vi "Main VI.vi"() -> ()   [LabVIEW 2020]
uses:
  Type Def - States Machine.ctl
  <vilib>/Instr/_visa.llb/VISA Configure Serial Port (Instr).vi
panel:
  in  "Start":bool
  in  "Bytes to read":u32
  out "Chart - Humidity":dbl(graph)
  out "Chart - Temperature":dbl(graph)
  in  "stop":bool
  in  "File Path":path
  in  "Time before receiving data (Seconds)":dbl
  out "Humidity (%)":dbl
  out "Temperature":dbl
  in  "Separator Term":string
  in  "Command Letter":string
  in  "Connection port":refnum<visa-resource-name>
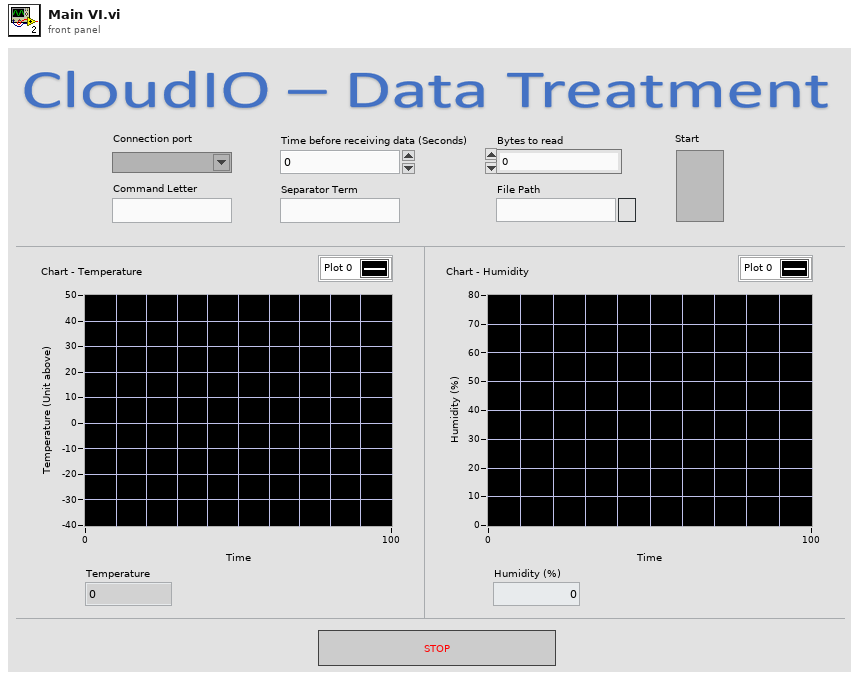
[diagram p1: front panel]
types:
  T1 = typedef "Type Def - States Machine.ctl" = enum16{"Idle", "Open Serial", "Request", "Receive", "Recording", "Close Serial"}
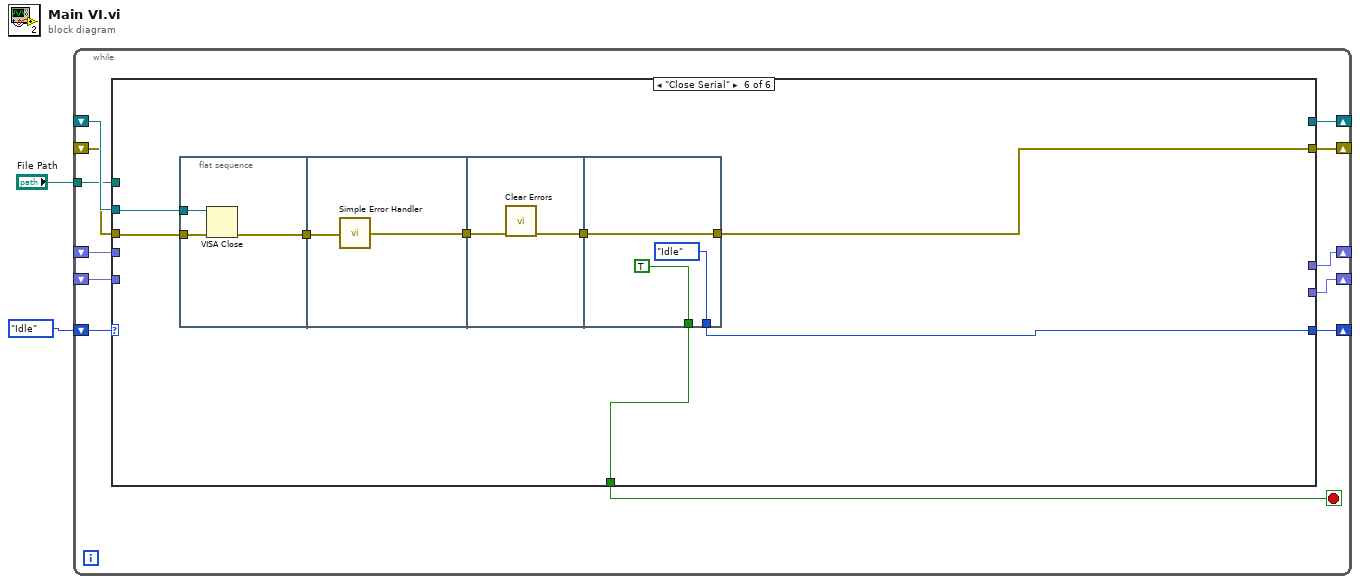
[diagram p0: block diagram]
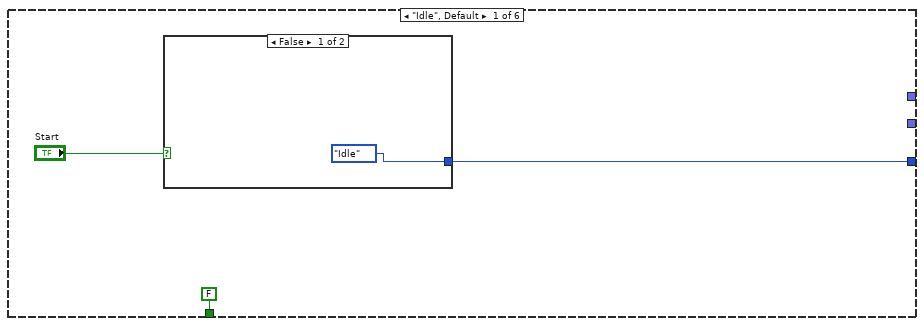
[diagram p2: hidden frame]
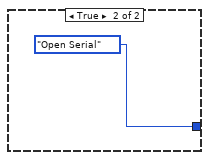
[diagram p3: hidden frame]
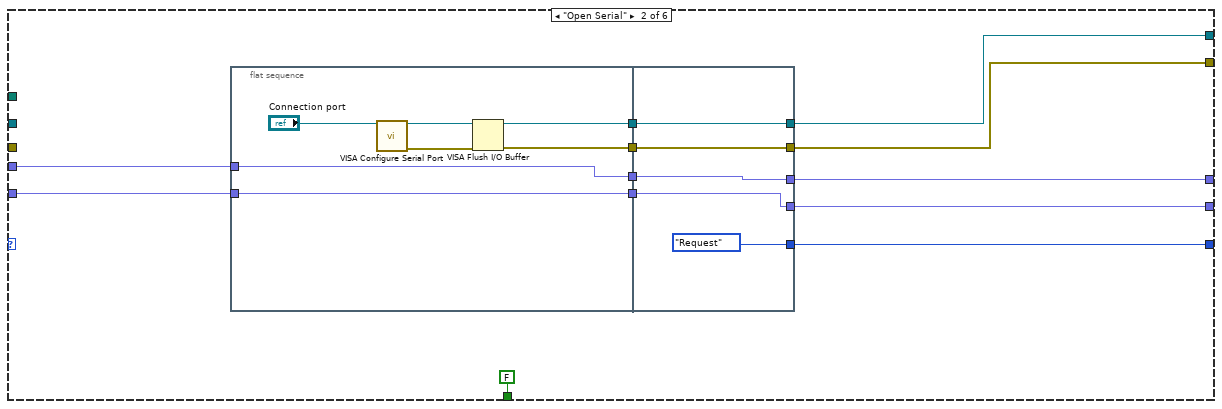
[diagram p4: hidden frame]
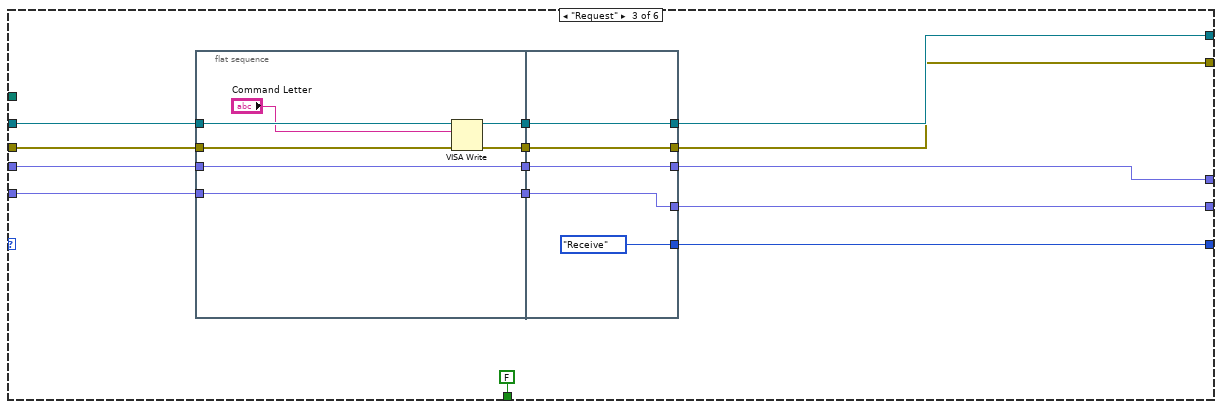
[diagram p5: hidden frame]
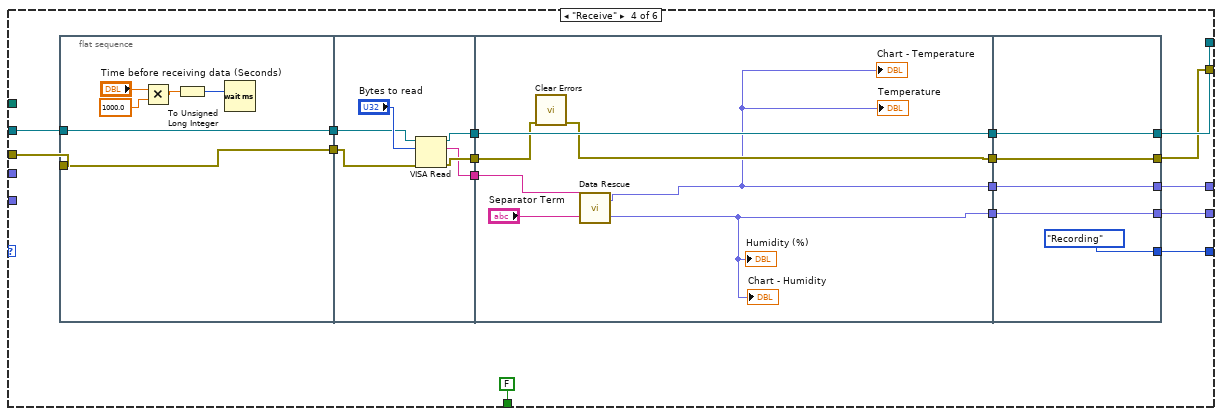
[diagram p6: hidden frame]
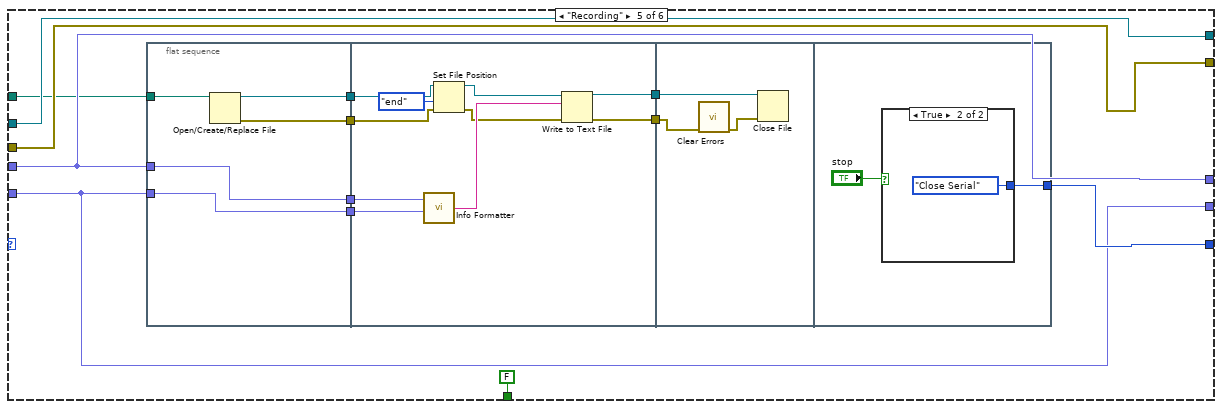
[diagram p7: hidden frame]
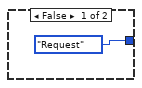
[diagram p8: hidden frame]
diagram:
  n1 = while {
    shift-right: [w11] -> _
    shift-left: Type_Def_-_States_Machine."Idle" ("Enum") -> [w14]
    shift-right: [w13] -> _
    shift-left: _ -> [w10]
    shift-right: [w12] -> _
    shift-left: _ -> [w9]
    shift-right: [w6] -> _
    shift-left: _ -> [w8]
    shift-right: [w7] -> _
    shift-left: _ -> [w5]
    tunnel: "File Path" -> [w3]
    stop <- w4 stop-if-true
    n2 = case shown="\"Close Serial\"" w14 {
      tunnel: [_ w31 w55 w85 w112 _] -> w13
      tunnel: [_ w29 w54 w70 w113 w149] -> w12
      tunnel: [w15 w27 w51 w78 w117 w146] -> w11
      tunnel: w10 -> [_ _ w57 w71 w112 w153]
      tunnel: w9 -> [_ _ w56 w86 w113 w152]
      tunnel: w8 -> [_ w23 w47 _ w115 _]
      tunnel: [_ w22 w46 w84 w114 _] -> w7
      tunnel: [_ w25 w49 w83 w115 _] -> w6
      tunnel: w5 -> [_ w20 w44 _ w114 _]
      tunnel: [FALSE FALSE FALSE FALSE FALSE w147] -> w4
      tunnel: w3 -> [_ _ _ _ w111 _]
      frame "Idle", Default {
        n3 = case shown="False" "Start" {
          tunnel: [Type_Def_-_States_Machine."Idle" ("Enum") Type_Def_-_States_Machine."Open Serial" ("Enum")] -> w15
          frame False {
          }
          frame True {
          }
        }
      }
      frame "Open Serial" {
        n4 = flat-sequence {
          tunnel: [w35] -> w30
          tunnel: [w34] -> w28
          tunnel: [w33] -> w24
          tunnel: w23 -> [w33]
          tunnel: [w32] -> w21
          tunnel: w20 -> [w32]
          tunnel: [w43] -> w31
          tunnel: w30 -> [w43]
          tunnel: [w42] -> w29
          tunnel: w28 -> [w42]
          tunnel: [Type_Def_-_States_Machine."Request" ("Enum")] -> w27
          tunnel: [w40] -> w25
          tunnel: w24 -> [w40]
          tunnel: [w39] -> w22
          tunnel: w21 -> [w39]
          frame #0 {
            n5 = call-poly "VISA Configure Serial Port"("VISA resource name"="Connection port") -> ("VISA resource name out"=w37:refnum<visa-resource-name>, "error out"=w38:errorcluster)  [unwired: 13 in]
            n6 = VISA Flush I/O Buffer(VISA resource name=w37, error in (no error)=w38) -> (VISA resource name out=w35:refnum<visa-resource-name>, error out=w34:errorcluster)  [unwired: 1 in]
          }
          frame #1 {
          }
        }
      }
      frame "Request" {
        n7 = flat-sequence {
          tunnel: [w61] -> w53
          tunnel: [w60] -> w52
          tunnel: [w59] -> w48
          tunnel: [w58] -> w45
          tunnel: w57 -> [w64]
          tunnel: w56 -> [w63]
          tunnel: w47 -> [w59]
          tunnel: w44 -> [w58]
          tunnel: [w68] -> w54
          tunnel: [w69] -> w55
          tunnel: w53 -> [w69]
          tunnel: w52 -> [w68]
          tunnel: [Type_Def_-_States_Machine."Receive" ("Enum")] -> w51
          tunnel: [w66] -> w49
          tunnel: w48 -> [w66]
          tunnel: [w65] -> w46
          tunnel: w45 -> [w65]
          frame #0 {
            n8 = VISA Write(VISA resource name=w64, write buffer="Command Letter", error in (no error)=w63) -> (VISA resource name out=w61:refnum<visa-resource-name>, error out=w60:errorcluster)  [unwired: 1 out]
          }
          frame #1 {
          }
        }
      }
      frame "Receive" {
        n9 = flat-sequence {
          tunnel: w86 -> [w91]
          tunnel: [w91] -> w73
          tunnel: [w92] -> w72
          tunnel: w71 -> [w92]
          tunnel: [w94] -> w76
          tunnel: [w96] -> w75
          tunnel: [w95] -> w74
          tunnel: w73 -> [w97]
          tunnel: w72 -> [w93]
          tunnel: w76 -> [w105]
          tunnel: w75 -> [w101]
          tunnel: w74 -> [w103]
          tunnel: [w105] -> w82
          tunnel: [w100] -> w81
          tunnel: [w102] -> w80
          tunnel: [w99] -> w79
          tunnel: [w107] -> w83
          tunnel: [w108] -> w84
          tunnel: [w109] -> w70
          tunnel: [w110] -> w85
          tunnel: w82 -> [w110]
          tunnel: w81 -> [w109]
          tunnel: w80 -> [w108]
          tunnel: w79 -> [w107]
          tunnel: [Type_Def_-_States_Machine."Recording" ("Enum")] -> w78
          frame #0 {
            n10 = Multiply(x="Time before receiving data (Seconds)", y=1000.0) -> (x*y=w90:dbl)
            n11 = To Unsigned Long Integer(number=w90) -> (unsigned 32bit integer=w88:u32)
            n12 = Wait (ms)(milliseconds to wait=w88) -> ()  [unwired: 1 out]
          }
          frame #1 {
            n13 = VISA Read(VISA resource name=w93, byte count="Bytes to read", error in (no error)=w97) -> (VISA resource name out=w94:refnum<visa-resource-name>, read buffer=w95:string, error out=w96:errorcluster)  [unwired: 1 out]
          }
          frame #2 {
            n14 = call <vilib>:"Clear Errors.vi"("error in (no error)"=w101) -> ("error out"=w100:errorcluster)  [unwired: 5 in, 1 out]
            n15 = call "Data Rescue.vi"("Separator"="Separator Term", "Input String"=w103) -> ("Humidity (%)"=w102:fxp<+/-,64,32>, "Temperature"=w99:fxp<+/-,64,32>)
            "Temperature" <- w99
            "Humidity (%)" <- w102
            "Chart - Humidity" <- w102
            "Chart - Temperature" <- w99
          }
          frame #3 {
          }
        }
      }
      frame "Recording" {
        n16 = flat-sequence {
          tunnel: w115 -> [w126]
          tunnel: w114 -> [w125]
          tunnel: [w128] -> w123
          tunnel: [w127] -> w122
          tunnel: [w126] -> w121
          tunnel: [w125] -> w120
          tunnel: w111 -> [w124]
          tunnel: w123 -> [w131]
          tunnel: w122 -> [w133]
          tunnel: w121 -> [w137]
          tunnel: w120 -> [w138]
          tunnel: [w135] -> w119
          tunnel: [w134] -> w118
          tunnel: w119 -> [w141]
          tunnel: w118 -> [w140]
          tunnel: [w142] -> w117
          frame #0 {
            n17 = Open/Create/Replace File(file path (use dialog)=w124) -> (refnum out=w127:refnum<file>, error out=w128:errorcluster)  [unwired: 5 in, 1 out]
          }
          frame #1 {
            n18 = call "Info Formatter.vi"("Humidity (%)"=w138, "Temperature (°C)"=w137) -> ("concatenated string"=w136:string)
            n19 = Set File Position(refnum=w133, from (0:start)=enum16{"start", "end", "current"}."end", error in=w131) -> (refnum out=w132:refnum<file>, error out=w130:errorcluster)  [unwired: 1 in]
            n20 = Write to Text File(file (use dialog)=w132, text=w136, error in=w130) -> (refnum out=w135:refnum<file>, error out=w134:errorcluster)  [unwired: 1 in, 1 out]
          }
          frame #2 {
            n21 = call <vilib>:"Clear Errors.vi"("error in (no error)"=w140) -> ("error out"=w139:errorcluster)  [unwired: 5 in, 1 out]
            n22 = Close File(refnum=w141, error in=w139) -> ()  [unwired: 2 out]
          }
          frame #3 {
            n23 = case shown="True" "stop" {
              tunnel: [Type_Def_-_States_Machine."Request" ("Enum") Type_Def_-_States_Machine."Close Serial" ("Enum")] -> w142
              frame False {
              }
              frame True {
              }
            }
          }
        }
      }
      frame "Close Serial" {
        n24 = flat-sequence {
          tunnel: w153 -> [w156]
          tunnel: w152 -> [w155]
          tunnel: [w154] -> w151
          tunnel: w151 -> [w158]
          tunnel: [w157] -> w150
          tunnel: w150 -> [w160]
          tunnel: [w159] -> w148
          tunnel: w148 -> [w163]
          tunnel: [TRUE] -> w147
          tunnel: [Type_Def_-_States_Machine."Idle" ("Enum")] -> w146
          tunnel: [w163] -> w149
          frame #0 {
            n25 = VISA Close(VISA resource name=w156, error in (no error)=w155) -> (error out=w154:errorcluster)
          }
          frame #1 {
            n26 = call <vilib>:"Simple Error Handler.vi"("error in (no error)"=w158) -> ("error out"=w157:errorcluster)  [unwired: 4 in, 4 out]
          }
          frame #2 {
            n27 = call <vilib>:"Clear Errors.vi"("error in (no error)"=w160) -> ("error out"=w159:errorcluster)  [unwired: 5 in, 1 out]
          }
          frame #3 {
          }
        }
      }
    }
  }
